vi "SMSSD.vi"() -> ()   [LabVIEW 2020]
uses:
  States.ctl
  <vilib>/ErrorRing/Error Ring.xnode
panel:
  out "SSD":T1
  in  "stop":bool
  in  "Number":u8
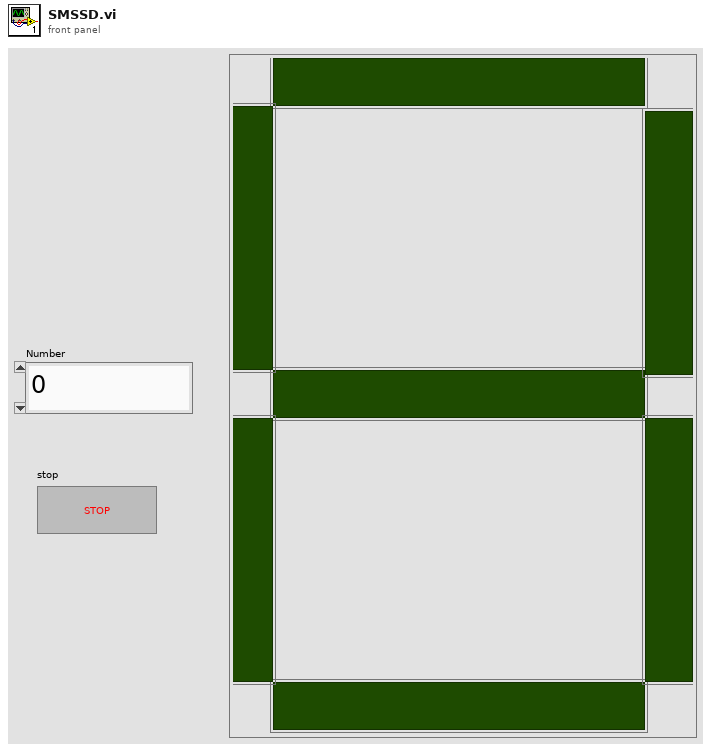
[diagram p1: front panel]
types:
  T1 = cluster{"a":bool, "g":bool, "d":bool, "f":bool, "b":bool, "c":bool, "e":bool}
  T2 = typedef "States.ctl" = enum16{"Idle", "UIInit", "DataInit", "NumToDisp", "UIUpdate", "Exit"}
  T3 = cluster{"TimeOut":i32, "Data":u8, "SSDDisp":cluster{"a":bool, "g":bool, "d":bool, "f":bool, "b":bool, "c":bool, "e":bool}}
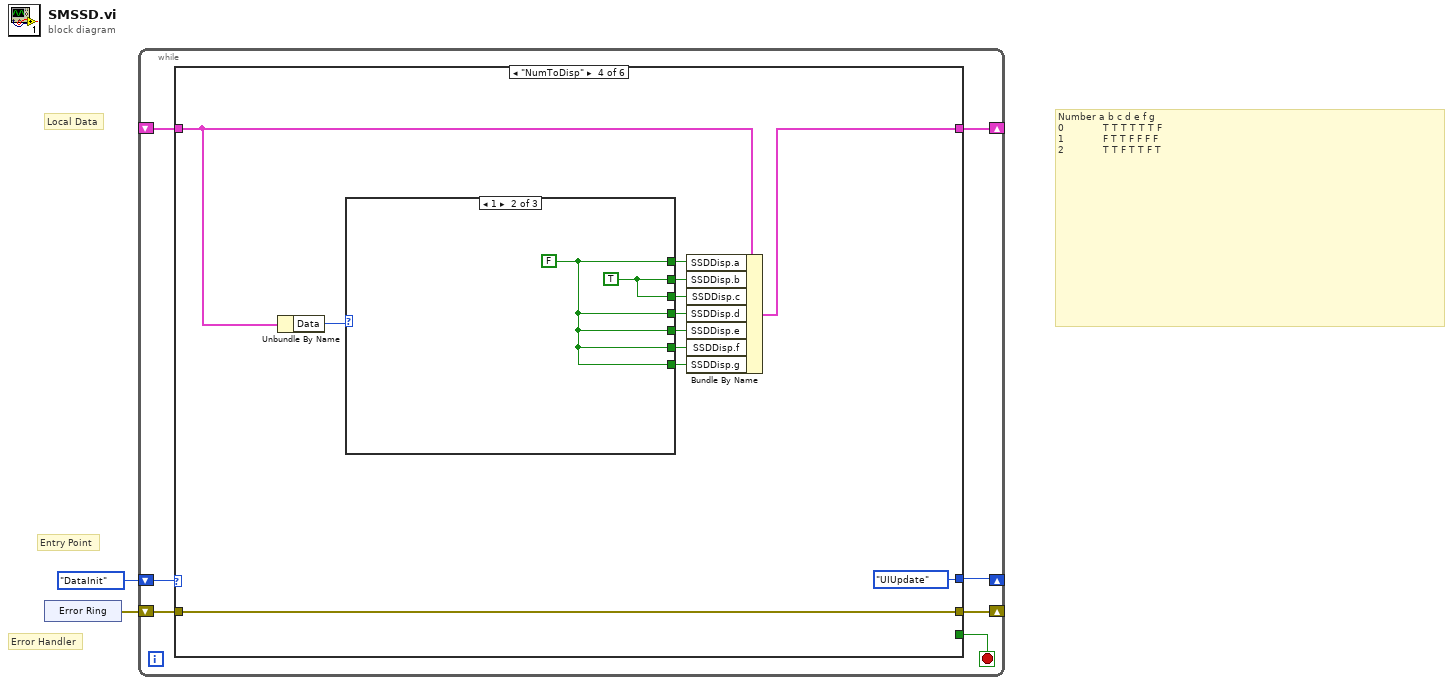
[diagram p0: block diagram]
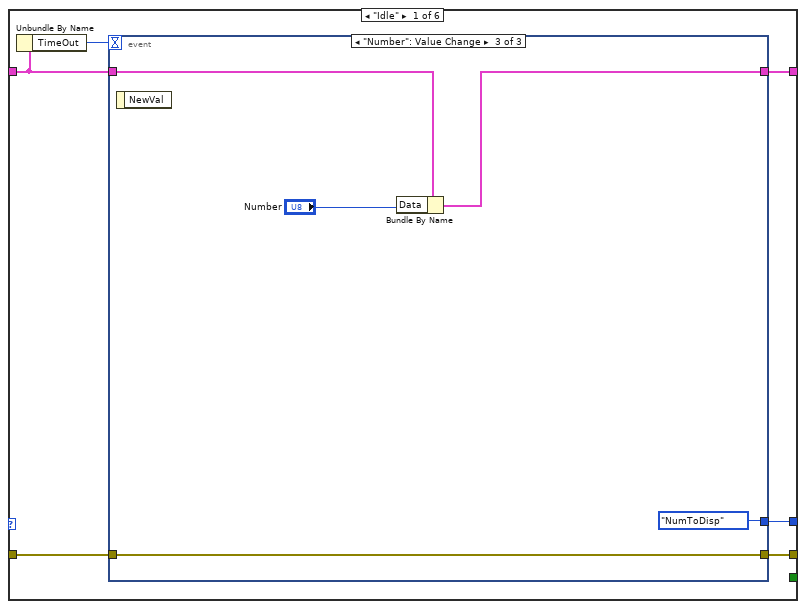
[diagram p2: hidden frame]
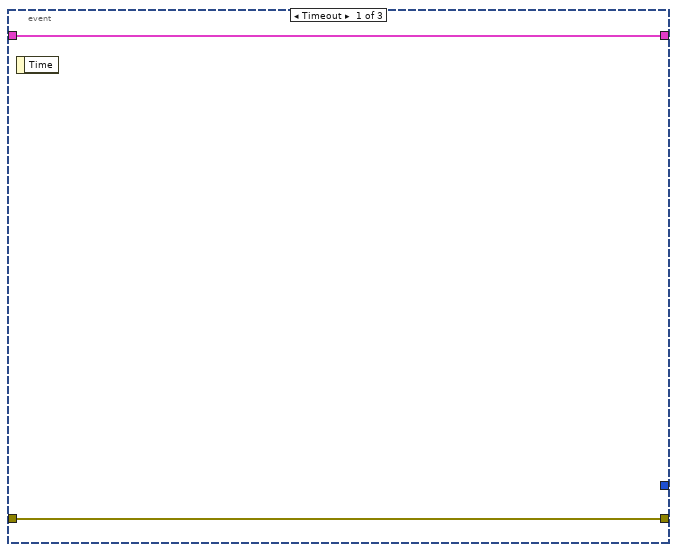
[diagram p3: hidden frame]
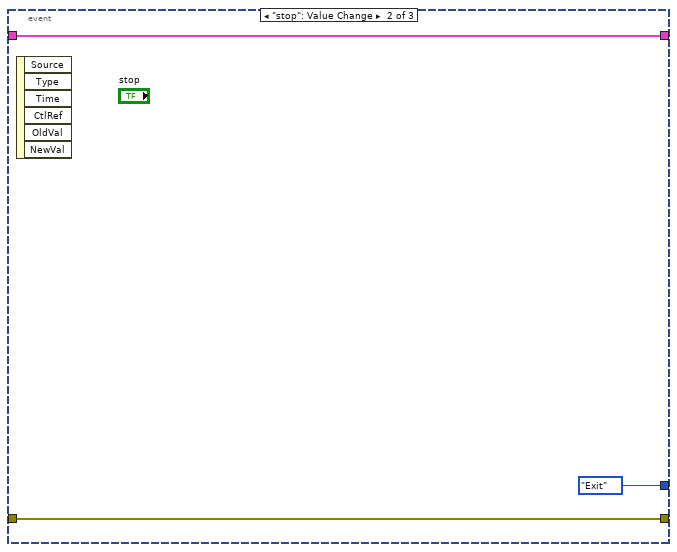
[diagram p4: hidden frame]
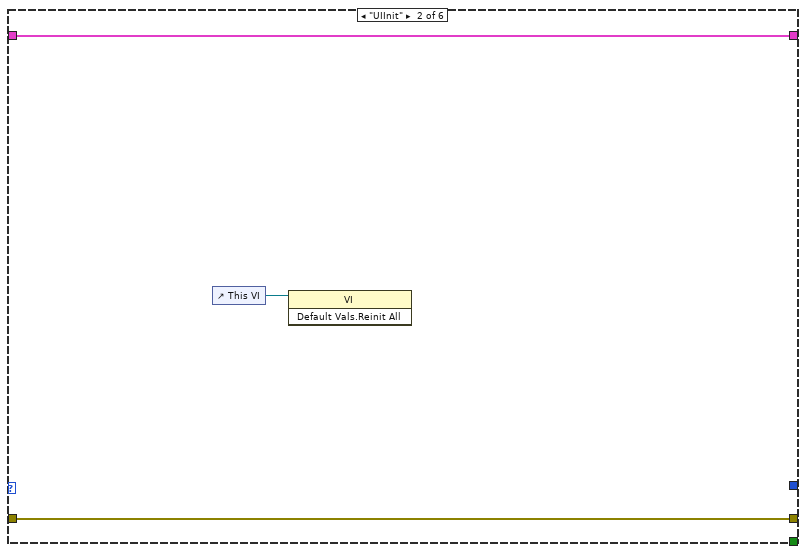
[diagram p5: hidden frame]
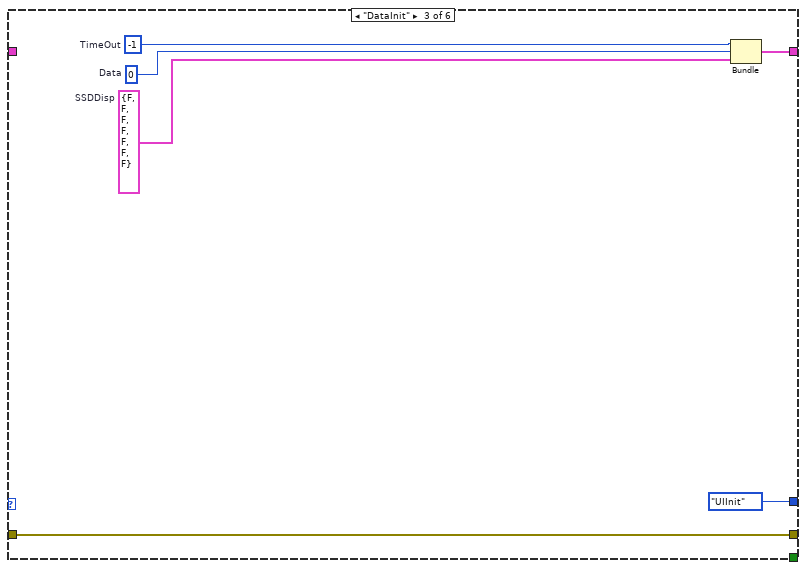
[diagram p6: hidden frame]
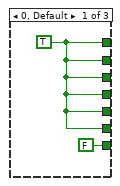
[diagram p7: hidden frame]
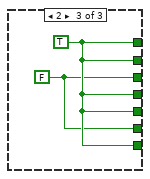
[diagram p8: hidden frame]
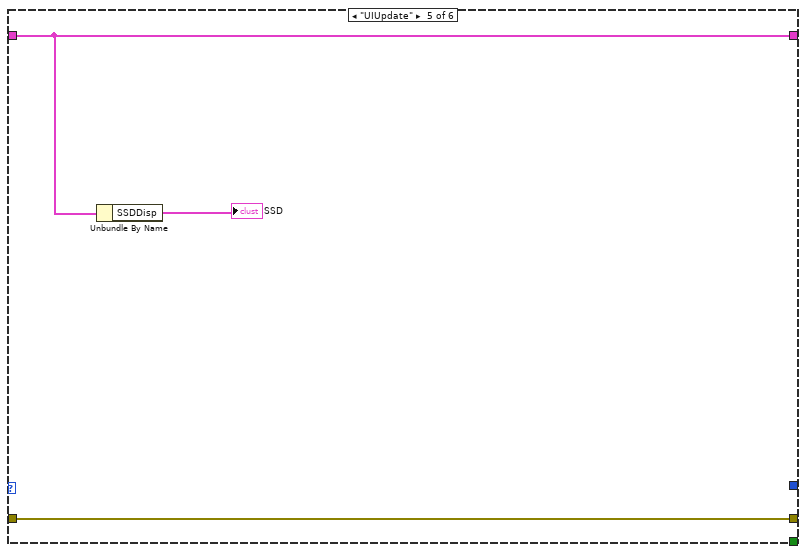
[diagram p9: hidden frame]
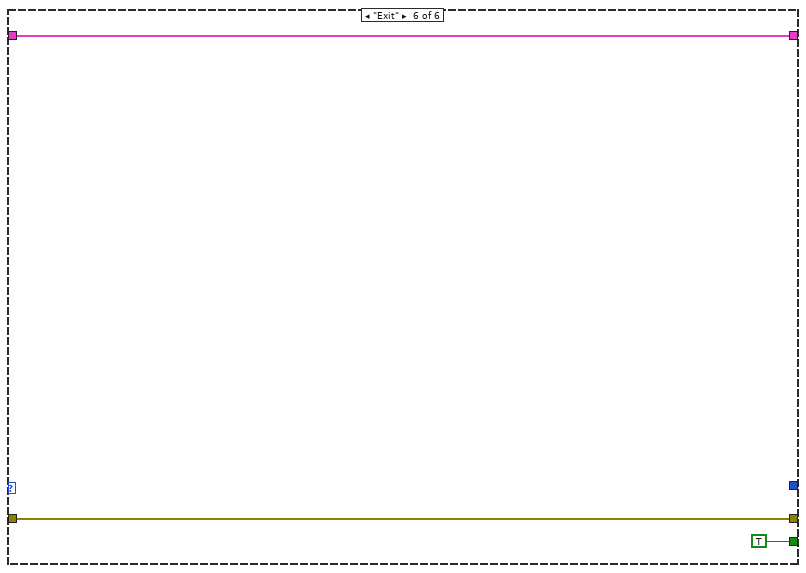
[diagram p10: hidden frame]
diagram:
  # "Number a b c d e f g\n0             T T T T T T F\n1             F T T F F F F\n2             T T F T T F T"
  # "Error Handler"
  # "Entry Point"
  # "Local Data"
  n1 = xnode "Error Ring"() -> ("error out"=w1:errorcluster)
  n2 = while {
    shift-right: [w4] -> _
    shift-left: States."DataInit" -> [w9]
    shift-right: [w7] -> _
    shift-left: w1 -> [w8]
    shift-right: [w6] -> _
    shift-left: _ -> [w5]
    stop <- w3 stop-if-true
    n3 = case shown="\"NumToDisp\"" w9 {
      tunnel: w8 -> [w15 w28 w34 w46 w55 w58]
      tunnel: [w14 w28 w34 w46 w55 w58] -> w7
      tunnel: [w13 w27 w32 w44 w54 w57] -> w6
      tunnel: w5 -> [w11 w27 _ w43 w54 w57]
      tunnel: [w12 _ States."UIInit" States."UIUpdate" _ _] -> w4
      tunnel: [_ _ _ _ _ TRUE] -> w3
      frame "Idle" {
        n4 = Unbundle By Name(w11) -> ("TimeOut"=w10:i32)
        n5 = event shown="[2] \"Number\": Value Change" {
          selector: _ -> [_ _ _]
          dyn-events: _ -> [_ _ _]
          timeout: w10 -> [_ _ _]
          tunnel: w15 -> [w17 w20 w25]
          tunnel: [w17 w20 w25] -> w14
          tunnel: w11 -> [w16 w19 w23]
          tunnel: [w16 w19 w24] -> w13
          tunnel: [_ States."Exit" States."NumToDisp"] -> w12
          event Timeout {
            n6 = event-data() -> ()  [unwired: 1 in, 1 out]
          }
          event "stop": Value Change {
            n7 = event-data() -> ()  [unwired: 1 in, 6 out]
          }
          event "Number": Value Change {
            n8 = event-data() -> ()  [unwired: 1 in, 1 out]
            n9 = Bundle By Name(cluster=w23, "Data"="Number") -> (w24:T3)
          }
        }
      }
      frame "UIInit" {
        n10 = control-ref of="This VI"() -> (w26:refnum<vi>)
        n11 = invoke class="VI" method="Default Vals.Reinit All"(reference=w26) -> ()  [unwired: 2 in, 3 out]
      }
      frame "DataInit" {
        w29 = T1 {"a"=FALSE, "g"=FALSE, "d"=FALSE, "f"=FALSE, "b"=FALSE, "c"=FALSE, "e"=FALSE}  # SSDDisp
        w31 = u8 0  # Data
        w33 = -1  # TimeOut
        n12 = Bundle("TimeOut"=w33, "Data"=w31, "SSDDisp"=w29) -> (w32:T3)  [unwired: 1 in]
      }
      frame "NumToDisp" {
        n13 = Unbundle By Name(w43) -> ("Data"=w45:u8)
        n14 = case shown="1" w45 {
          tunnel: [w48 w49 w52] -> w41
          tunnel: [w48 w50 w52] -> w40
          tunnel: [w48 w50 w51] -> w39
          tunnel: [w48 w49 w52] -> w38
          tunnel: [w48 w49 w52] -> w37
          tunnel: [w48 w49 w51] -> w36
          tunnel: [FALSE w49 w52] -> w35
          frame 0, Default {
            w48 = TRUE
          }
          frame 1 {
            w49 = FALSE
            w50 = TRUE
          }
          frame 2 {
            w51 = FALSE
            w52 = TRUE
          }
        }
        n15 = Bundle By Name(cluster=w43, "SSDDisp.a"=w41, "SSDDisp.b"=w40, "SSDDisp.c"=w39, "SSDDisp.d"=w38, "SSDDisp.e"=w37, "SSDDisp.f"=w36, "SSDDisp.g"=w35) -> (w44:T3)
      }
      frame "UIUpdate" {
        n16 = Unbundle By Name(w54) -> ("SSDDisp"=→"SSD":T1)
      }
      frame "Exit" {
      }
    }
  }
